vi "example test.vi"() -> (0 "input error":errorcluster, 1 "input lookup error":errorcluster, 2 "init error":errorcluster, 3 "correct execution settings":bool, 4 "no data written":bool, 5 "output lookup error":errorcluster, 6 "output error":errorcluster, 7 "serialization problem":errorcluster, 8 "final error":errorcluster, 11 "invalid configuration":errorcluster)   [LabVIEW 2020, in "dds tests.lvlib"]
uses:
  dds tests.lvlib
  module/configuration/dds configuration.lvclass
  <vilib>/NI/Tag Bus Module Framework/channel/TBM channel.lvclass
  <vilib>/NI/Tag Bus/tag/Data Type.ctl
  <vilib>/NI/Tag Bus/tag/tag descriptor.lvclass
  <vilib>/NI/Tag Bus Module Framework/channel/channel classification.ctl
  module/execution/dds runtime.lvclass
  <vilib>/NI/Tag Bus/dictionary/data dictionary.lvclass
  <vilib>/NI/Tag Bus/dictionary/lookup polymorphs/locate double.vi
  <vilib>/NI/Tag Bus/table/data table.lvlib
  <vilib>/NI/Tag Bus/table/data polymorphs/write one/write Double.vi
  <vilib>/NI/Configuration Framework/serializable configuration/NISE_CEF_serializable configuration.lvclass
  <vilib>/RTI DDS Toolkit/Types/RTI DDS Advanced Reader Configuration.ctl
  <vilib>/RTI DDS Toolkit/Library/LVDDS_library.lvlib
  module/configuration/Line.ctl
  <vilib>/NI/Tag Bus/table/data polymorphs/read one/read Double.vi
  C:/Program Files (x86)/National Instruments/LabVIEW 2020/vi.lib/NI/Tag Bus Module Framework/module configuration/TBM module configuration.lvclass
  C:/Program Files (x86)/National Instruments/LabVIEW 2020/vi.lib/NI/Tag Bus Module Framework/root configuration/TBM configuration.lvclass
  C:/Program Files (x86)/National Instruments/LabVIEW 2020/vi.lib/NI/Configuration Framework/serializable configuration/NISE_CEF_serializable configuration.lvclass
  C:/Users/u386974/Documents/user.lib/LV2020/DDS/source/module/configuration/dds configuration.lvclass
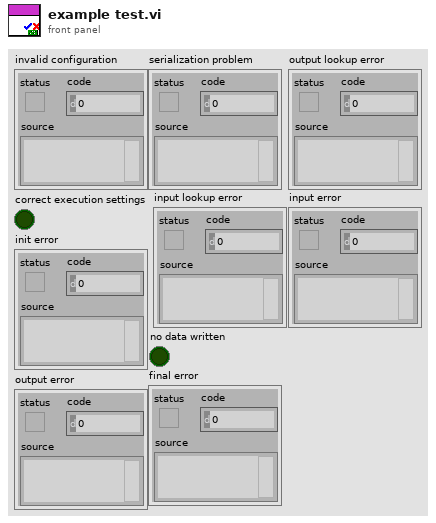
[diagram p1: front panel]
types:
  T1 = typedef "DDS configuration.lvclass/Line.ctl" = cluster{"channel":refnum<class "TBM channel.lvclass">, "DDS topic":string, "DDS Domain":u32, "advanced configuration":T2}
  T2 = typedef "LVDDS_library.lvlib/RTI DDS Advanced Reader Configuration.ctl" = cluster{"typeName":string, "keyName":string, "domainParticipantQoSProfile":string, "dataReaderQoSProfile":string, "forceArrayMapping?":bool, "forceExclusiveReader?":bool, "forceRead? (only ExclusiveReader)":bool, "forceUnboundedString?":bool}
  T3 = typedef "TBM channel.lvclass/channel classification.ctl" = enum16{"input data", "output data", "processing parameter", "processing result"}
  T4 = typedef "tag bus.lvlib/tag descriptor.lvclass/Data Type.ctl" = enum16{"Double", "Single", "I64", "I32", "I16", "I8", "U64", "U32", "U16", "U8", "Boolean", "String", "Array of Double", "Array of Single", "Array of I64", "Array of I32", "Array of I16", "Array of I8", "Array of U64", "Array of U32", "Array of U16", "Array of U8", "Array of Boolean", "Array of String"}
  T5 = typedef "TBM channel.lvclass/data tables.ctl" = cluster{"input data":T6, "processing parameter":T6, "processing result":T6, "output data":T6}
  T6 = typedef "tag bus.lvlib/dictionary table pair.ctl" = cluster{"data dictionary":refnum<class "data dictionary.lvclass">, "data table":T7}
  T7 = typedef "tag bus.lvlib/data table.lvlib/data table.ctl" = cluster{"Double":dbl[], "Single":sgl[], "I64":i64[], "I32":i32[], "I16":i16[], "I8":i8[], "U64":u64[], "U32":u32[], "U16":u16[], "U8":u8[], "Boolean":bool[], "String":string[], "Array of Double":cluster{"DBL Array":dbl[]}[], "Array of Single":cluster{"SGL Array":sgl[]}[], "Array of I64":cluster{"I64 Array":i64[]}[], "Array of I32":cluster{"I32 Array":i32[]}[], "Array of I16":cluster{"I16 Array":i16[]}[], "Array of I8":cluster{"I8 Array":i8[]}[], "Array of U64":cluster{"U64 Array":u64[]}[], "Array of U32":cluster{"U32 Array":u32[]}[], "Array of U16":cluster{"U16 Array":u16[]}[], "Array of U8":cluster{"U8 Array":u8[]}[], "Array of Boolean":cluster{"Boolean Array":bool[]}[], "Array of String":cluster{"String Array":string[]}[]}
  T8 = typedef "TBM module execution interface.lvclass/execution settings.ctl" = cluster{"reads inputs":bool, "processes data":bool, "writes outputs":bool}
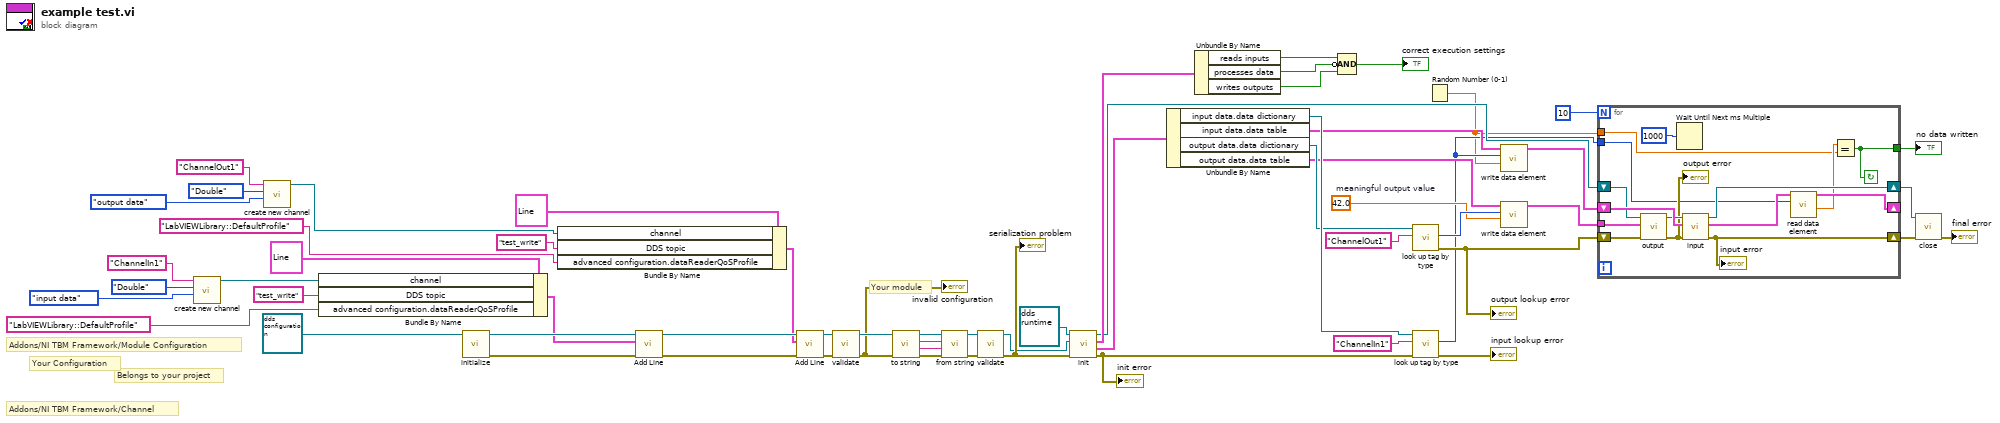
[diagram p0: block diagram]
diagram:
  w28 = 42.0  # meaningful output value
  # "Your module"
  # "Your Configuration"
  # "Addons/NI TBM Framework/Module Configuration"
  # "Belongs to your project"
  # "Addons/NI TBM Framework/Channel"
  n1 = call <vilib>:"create new channel.vi"("channel classification"=channel_classification."input data", "data type"=Data_Type."Double", "channel name"="ChannelIn1") -> ("channel"=w12:refnum<class "TBM channel.lvclass">)  [unwired: 8 in]
  n2 = call <vilib>:"create new channel.vi"("channel classification"=channel_classification."output data", "data type"=Data_Type."Double", "channel name"="ChannelOut1") -> ("channel"=w18:refnum<class "TBM channel.lvclass">)  [unwired: 8 in]
  n3 = Bundle By Name(cluster=T1 {"channel"=refnum, "DDS topic"="", "DDS Domain"=0, "advanced configuration"={"typeName"="", "keyName"="", "domainParticipantQoSProfile"="", "dataReaderQoSProfile"="", "forceArrayMapping?"=FALSE, "forceExclusiveReader?"=FALSE, "forceRead? (only ExclusiveReader)"=FALSE, "forceUnboundedString?"=FALSE}} ("Line"), "channel"=w12, "DDS topic"="test_write", "advanced configuration.dataReaderQoSProfile"="LabVIEWLibrary::DefaultProfile") -> (w13:T1)
  n4 = call <vilib>:"initialize.vi"("configuration in"=refnum<class "dds configuration.lvclass"> refnum ("tag bus configurable plugin module configuration")) -> ("error out"=w20:errorcluster, "configuration out"=w21:refnum<class "dds configuration.lvclass">)  [unwired: 8 in, 1 out]
  n5 = Bundle By Name(cluster=T1 {"channel"=refnum, "DDS topic"="", "DDS Domain"=0, "advanced configuration"={"typeName"="", "keyName"="", "domainParticipantQoSProfile"="", "dataReaderQoSProfile"="", "forceArrayMapping?"=FALSE, "forceExclusiveReader?"=FALSE, "forceRead? (only ExclusiveReader)"=FALSE, "forceUnboundedString?"=FALSE}} ("Line"), "channel"=w18, "DDS topic"="test_write", "advanced configuration.dataReaderQoSProfile"="LabVIEWLibrary::DefaultProfile") -> (w17:T1)
  n6 = call "Add Line.vi"("error in"=w20, "Line"=w13, "dds configuration in"=w21) -> ("error out"=w22:errorcluster, "dds configuration out"=w24:refnum<class "dds configuration.lvclass">)  [unwired: 7 in]
  n7 = call "Add Line.vi"("error in"=w22, "Line"=w17, "dds configuration in"=w24) -> ("error out"=w19:errorcluster, "dds configuration out"=w23:refnum<class "dds configuration.lvclass">)  [unwired: 7 in]
  n8 = call-dynamic "validate.vi"("error in"=w19, "dds configuration in"=w23) -> ("error out"=w54:errorcluster, "dds configuration out"=w55:refnum<class "dds configuration.lvclass">)  [unwired: 8 in]
  "invalid configuration" <- w54
  n9 = call-dynamic "to string.vi"("error in"=w54, "dds configuration in"=w55) -> ("error out"=w50:errorcluster, "data"=w51:string, "version"=w52:string, "dds configuration out"=w53:refnum<class "dds configuration.lvclass">)  [unwired: 6 in]
  n10 = call-dynamic "from string.vi"("error in"=w50, "data"=w51, "version"=w52, "dds configuration in"=w53) -> ("error out"=w48:errorcluster, "dds configuration out"=w49:refnum<class "dds configuration.lvclass">)  [unwired: 6 in]
  n11 = call-dynamic "validate.vi"("error in"=w48, "dds configuration in"=w49) -> ("error out"=w46:errorcluster, "dds configuration out"=w45:refnum<class "dds configuration.lvclass">)  [unwired: 8 in]
  "serialization problem" <- w46
  n12 = call-dynamic "init.vi"("error in"=w46, "TBM module configuration in"=w45, "dds runtime in"=refnum<class "dds runtime.lvclass"> refnum ("tag bus configurable plugin module")) -> ("error out"=w37:errorcluster, "data allocations"=w39:T5, "execution settings"=w44:T8, "dds runtime out"=w6:refnum<class "dds runtime.lvclass">)  [unwired: 5 in]
  "init error" <- w37
  n13 = Unbundle By Name(w39) -> ("input data.data dictionary"=w38:refnum<class "data dictionary.lvclass">, "input data.data table"=w35:T7, "output data.data dictionary"=w32:refnum<class "data dictionary.lvclass">, "output data.data table"=w29:T7)
  n14 = Unbundle By Name(w44) -> ("reads inputs"=w41:bool, "processes data"=w43:bool, "writes outputs"=w42:bool)
  n15 = Compound Arithmetic op=AND(w41, invert w43, w42) -> (→"correct execution settings":bool)
  n16 = call-poly <vilib>:"look up tag by type.vi"("name"="ChannelOut1" ("channel name"), "data dictionary in"=w32) -> ("error out"=w8:errorcluster, "index"=w30:i32)  [unwired: 7 in, 1 out]
  "output lookup error" <- w8
  n17 = call-poly <vilib>:"look up tag by type.vi"("error in"=w37, "name"="ChannelIn1" ("channel name"), "data dictionary in"=w38) -> ("error out"=→"input lookup error":errorcluster, "index"=w3:i32)  [unwired: 6 in, 1 out]
  n18 = Random Number (0-1)() -> (number: 0 to 1=w2:dbl)
  n19 = call-poly <vilib>:"write data element.vi"("value"=w2, "index"=w3, "data table in"=w35) -> ("data table out"=w33:T7)  [unwired: 8 in]
  n20 = call-poly <vilib>:"write data element.vi"("value"=w28, "index"=w30, "data table in"=w29) -> ("data table out"=w27:T7)  [unwired: 8 in]
  n21 = for {
    N: 10 -> [_]
    tunnel: w27 -> [w75]
    shift-right: [w66] -> _
    shift-left: w33 -> [w76]
    shift-right: [w69] -> w5
    shift-left: w8 -> [w74]
    shift-right: [w71] -> w7
    shift-left: w6 -> [w70]
    tunnel: w3 -> [w65]
    tunnel: w2 -> [w63]
    tunnel: [w62] -> w1
    stop <- w62 continue-if-true
    n22 = call-dynamic "output.vi"("error in"=w74, "data table in"=w75, "dds runtime in"=w70) -> ("error out"=w72:errorcluster, "dds runtime out"=w73:refnum<class "dds runtime.lvclass">)  [unwired: 6 in, 1 out]
    "output error" <- w72
    n23 = Wait Until Next ms Multiple(millisecond multiple=u32 1000) -> ()  [unwired: 1 out]
    n24 = call-dynamic "input.vi"("error in"=w72, "data table in"=w76, "dds runtime in"=w73) -> ("error out"=w69:errorcluster, "data table out"=w67:T7, "dds runtime out"=w71:refnum<class "dds runtime.lvclass">)  [unwired: 6 in]
    "input error" <- w69
    n25 = call-poly <vilib>:"read data element.vi"("index"=w65, "data table in"=w67) -> ("value"=w64:dbl, "data table out"=w66:T7)  [unwired: 8 in]
    n26 = Equal?(x=w64, y=w63) -> (x = y?=w62:bool)
  }
  "no data written" <- w1
  n27 = call-dynamic "close.vi"("error in"=w5, "dds runtime in"=w7) -> ("error out"=→"final error":errorcluster)  [unwired: 9 in]
